vi "Server_State.vi"(8 "error in (no error)":errorcluster, 11 "Server":path) -> (0 "error out":errorcluster, 1 "Connected?":bool, 3 "Connection":string)   [LabVIEW 2020]
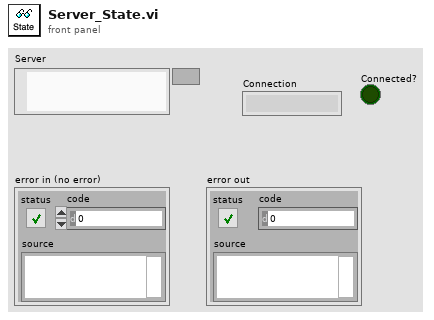
[diagram p1: front panel]
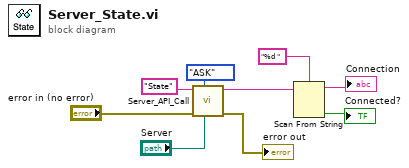
[diagram p0: block diagram]
diagram:
  n1 = call "Server_API_Call.vi"("Server"="Server", "Direction"=enum16{"ASK", "TELL"}."ASK", "error in (no error)"="error in (no error)", "cmd"="State" ("url")) -> ("error out"=→"error out":errorcluster, "Read from Server"=w4:string)  [unwired: 5 in, 1 out]
  n2 = Scan From String(format string="%d ", input string=w4) -> (remaining string=→"Connection":string, output 1=→"Connected?":bool)  [unwired: 3 in, 2 out]
